vi "Calibrate Laser Diode.vi"(0 "COM Port in":refnum<visa-resource-name>, 1 "error in":errorcluster) -> (2 "COM Port out":refnum<visa-resource-name>, 3 "OK":bool, 4 "error out":errorcluster)   [LabVIEW 2013]
doc: "This command recalibrates the laser diode because of aging issues.\n\nPlease start calibration only if the laser shows a significant power drop.\n\nIf the laser does not achieve its specified laser power because of aging issues recalibrating\nwill compensate the power drop by recalculating the maximum diode current and bias offset.\n\nCAUTION: during the calibration progress the laser will emit laser light."
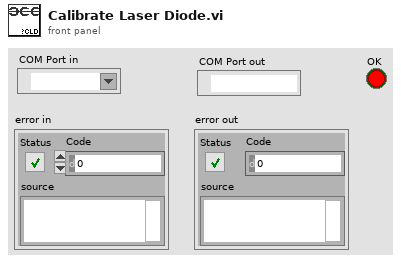
[diagram p1: front panel]
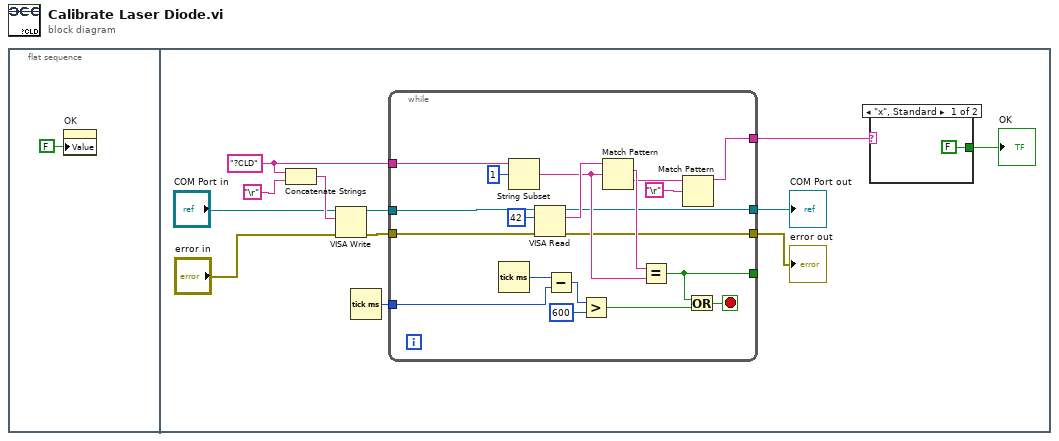
[diagram p0: block diagram]
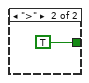
[diagram p2: hidden frame]
diagram:
  n1 = flat-sequence {
    frame #0 {
      n2 = property on="OK" class="Bool. (strikt)"("Value"=FALSE ("OK")) -> ()  [unwired: 2 in, 2 out]
    }
    frame #1 {
      w5 = "?CLD" ("Schreibpuffer")
      n3 = Concatenate Strings(w5, "\r") -> (w11:string)
      n4 = VISA Write(VISA resource name="COM Port in", write buffer=w11, error in (no error)="error in") -> (VISA resource name out=w7:refnum<visa-resource-name>, error out=w6:errorcluster)  [unwired: 1 out]
      n5 = Tick Count (ms)() -> (millisecond timer value=w4:u32)
      n6 = while {
        tunnel: [w30] -> w13
        tunnel: [w29] -> w12
        tunnel: [w28] -> w3
        tunnel: [w24] -> _
        tunnel: w7 -> [w17]
        tunnel: w6 -> [w26]
        tunnel: w5 -> [w25]
        tunnel: w4 -> [w21]
        stop <- w23 stop-if-true
        n7 = Tick Count (ms)() -> (millisecond timer value=w22:u32)
        n8 = String Subset(string=w25, offset (0)=1 ("Offset (0)")) -> (substring=w31:string)  [unwired: 1 in]
        n9 = VISA Read(VISA resource name=w17, byte count=u32 42 ("Byte-Anzahl"), error in (no error)=w26) -> (VISA resource name out=w30:refnum<visa-resource-name>, read buffer=w34:string, error out=w29:errorcluster)  [unwired: 1 out]
        n10 = Subtract(x=w22, y=w21) -> (x-y=w20:u32)
        n11 = Greater?(x=w20, y=u32 600) -> (0:w18:bool)
        n12 = Match Pattern(string=w34, regular expression=w31) -> (match substring=w33:string, after substring=w27:string)  [unwired: 1 in, 2 out]
        n13 = Equal?(x=w33, y=w31) -> (x = y?=w24:bool)
        n14 = Match Pattern(string=w27, regular expression="\r") -> (before substring=w28:string)  [unwired: 1 in, 3 out]
        n15 = Or(x=w24, y=w18) -> (x .or. y?=w23:bool)
      }
      "COM Port out" <- w13
      "error out" <- w12
      n16 = case shown="\"x\", Standard" w3 {
        tunnel: [FALSE TRUE] -> w2
        frame "x", Default {
        }
        frame ">" {
        }
      }
      "OK" <- w2
    }
  }
